vi "Unit Test Commands.vi"() -> ()   [LabVIEW 2015, in "Gas.lvclass"]
uses:
  Gas.lvclass
  Typedefs/Valves.ctl
  Typedefs/Pressure Sensor.ctl
panel:
  out "x = y?":bool[](array[boolean])
  out "Numeric 2":dbl
  out "Numeric":dbl
  out "time stamp":timestamp
  out "Mfg Serial Number":string
  out "Pressure":dbl
  out "Write Success?":bool
  out "Chemical Trap Success?":bool
  out "Heater Success?":bool
  out "Pump Success?":bool
  out "Valve Success?":bool
  out "Serial Number":string
  out "Hardware":string
  out "Firmware":string
  out "Ready?":bool
  out "error out":errorcluster
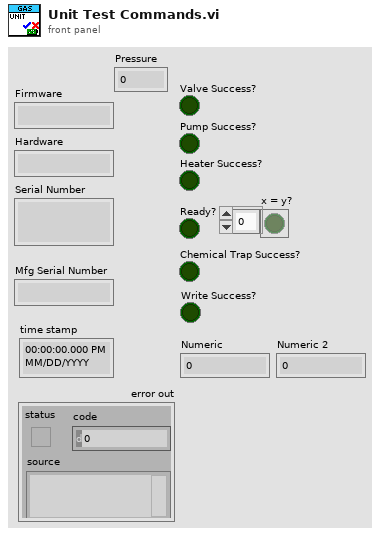
[diagram p1: front panel]
types:
  T1 = typedef "Gas.lvclass/Pressure Sensor.ctl" = u16
  T2 = typedef "Gas.lvclass/Valves.ctl" = u16
  T3 = typedef "Gas.lvclass/Session Handle.ctl" = refnum<data-value>
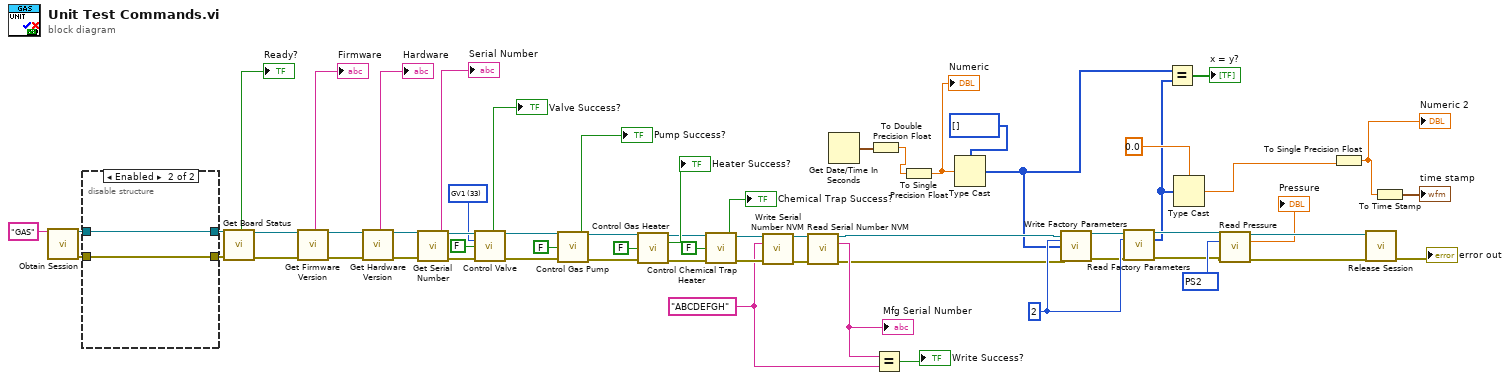
[diagram p0: block diagram]
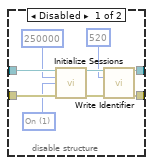
[diagram p2: hidden frame]
diagram:
  w15 = u8 2 ("Address")
  w20 = T1 225 items=["PS1"=224, "PS2"=225] ("Pressure Sensor")
  w22 = "ABCDEFGH" ("Serial Number")
  w39 = T2 33 items=["GV1"=33, "GV2"=34, "GV3"=35, "GV4"=36, "GV5"=37, "GV6"=38, "GV7"=39, "GV8"=40, "GV9"=41, "GV10"=42, "GV11"=43, "LV3"=51, "LV4"=52] ("Valves")
  n1 = call "Obtain Session.vi"("Session  Name ()"="GAS") -> ("Session Handle"=w62:T3, "error out"=w61:errorcluster)  [unwired: 13 in]
  n2 = disable-structure shown="Enabled" {
    disable-tunnel: w62 -> [w71 w73]
    disable-tunnel: w61 -> [w70 w72]
    disable-tunnel: [w64 w73] -> w59
    disable-tunnel: [w63 w72] -> w58
    frame Disabled {
      w68 = u32 1 items=["Off", "On"] ("Termination")
      n3 = call "Initialize Sessions.vi"("Session Handle in"=w71, "Baud Rate"=u32 250000, "Termination"=w68, "error in (no error)"=w70) -> ("Session Handle Out"=w67:T3, "error out"=w66:errorcluster)  [unwired: 10 in]
      n4 = call "Write Identifier.vi"("Session Handle in"=w67, "identifier"=u16 520, "error in (no error)"=w66) -> ("Session Handle out"=w64:T3, "error out"=w63:errorcluster)  [unwired: 11 in]
    }
    frame Enabled {
    }
  }
  n5 = call "Get Board Status.vi"("Session Handle in"=w59, "error in (no error)"=w58) -> ("Session Handle out"=w55:T3, "Ready?"=→"Ready?":bool, "error out"=w56:errorcluster)  [unwired: 11 in]
  n6 = call "Get Firmware Version.vi"("Session Handle in"=w55, "error in (no error)"=w56) -> ("Session Handle out"=w48:T3, "Firmware Version"=→"Firmware":string, "error out"=w49:errorcluster)  [unwired: 11 in]
  n7 = call "Get Hardware Version.vi"("Session Handle in"=w48, "error in (no error)"=w49) -> ("Session Handle out"=w46:T3, "Hardware Version"=→"Hardware":string, "error out"=w45:errorcluster)  [unwired: 11 in]
  n8 = call "Get Serial Number.vi"("Session Handle in"=w46, "error in (no error)"=w45) -> ("Session Handle out"=w42:T3, "Serial Number"=→"Serial Number":string, "error out"=w43:errorcluster)  [unwired: 11 in]
  n9 = call "Control Valve.vi"("Session Handle in"=w42, "Valves"=w39, "Energize?"=FALSE, "error in (no error)"=w43) -> ("Session Handle out"=w38:T3, "Success?"=→"Valve Success?":bool, "error out"=w37:errorcluster)  [unwired: 9 in]
  n10 = call "Control Gas Pump.vi"("Session Handle in"=w38, "On?"=FALSE, "error in (no error)"=w37) -> ("Session Handle out"=w34:T3, "Success?"=→"Pump Success?":bool, "error out"=w33:errorcluster)  [unwired: 10 in]
  n11 = call "Control Gas Heater.vi"("Session Handle in"=w34, "On?"=FALSE, "error in (no error)"=w33) -> ("Session Handle out"=w30:T3, "Success?"=→"Heater Success?":bool, "error out"=w29:errorcluster)  [unwired: 10 in]
  n12 = call "Control Chemical Trap Heater.vi"("Session Handle in"=w30, "On?"=FALSE, "error in (no error)"=w29) -> ("Session Handle out"=w23:T3, "Success?"=→"Chemical Trap Success?":bool, "error out"=w24:errorcluster)  [unwired: 10 in]
  n13 = call "Write Serial Number NVM.vi"("Session Handle in"=w23, "Serial Number"=w22, "error in (no error)"=w24) -> ("Session Handle out"=w26:T3, "error out"=w25:errorcluster)  [unwired: 11 in]
  n14 = call "Read Serial Number NVM.vi"("Session Handle in"=w26, "error in (no error)"=w25) -> ("Session Handle out"=w12:T3, "Serial Number"=w21:string, "error out"=w11:errorcluster)  [unwired: 11 in]
  "Mfg Serial Number" <- w21
  n15 = Get Date/Time In Seconds() -> (seconds since 1Jan1904=w8:timestamp)
  n16 = To Double Precision Float(number=w8) -> (double precision float=w9:dbl)
  n17 = Equal?(x=w21, y=w22) -> (x = y?=→"Write Success?":bool)
  n18 = To Single Precision Float(number=w9) -> (single precision float=w7:sgl)
  "Numeric" <- w7
  n19 = Type Cast(type=u8[] [], x=w7) -> (*(type *) &x=w3:u8[])
  n20 = call "Write Factory Parameters.vi"("Session Handle in"=w12, "Address"=w15, "Bytes to Write"=w3, "error in (no error)"=w11) -> ("Session Handle out"=w14:T3, "error out"=w13:errorcluster)  [unwired: 10 in]
  n21 = call "Read Factory Parameters.vi"("Session Handle in"=w14, "Address"=w15, "error in (no error)"=w13) -> ("Session Handle out"=w18:T3, "Read Bytes"=w4:u8[], "error out"=w17:errorcluster)  [unwired: 10 in]
  n22 = Equal?(x=w3, y=w4) -> (x = y?=→"x = y?":bool[])
  n23 = Type Cast(type=sgl 0.0, x=w4) -> (*(type *) &x=w1:sgl)
  n24 = call "Read Pressure.vi"("Session Handle in"=w18, "Pressure Sensor"=w20, "error in (no error)"=w17) -> ("Session Handle out"=w51:T3, "Pressure"=→"Pressure":dbl, "error out"=w52:errorcluster)  [unwired: 10 in]
  n25 = To Single Precision Float(number=w1) -> (single precision float=w5:sgl)
  "Numeric 2" <- w5
  n26 = call "Release Session.vi"("Session Handle"=w51, "error in (no error)"=w52) -> ("error out"=→"error out":errorcluster)  [unwired: 13 in]
  n27 = To Time Stamp(1:w5) -> (0:→"time stamp":timestamp)
